vi "Tokenize Statement.vi"(8 "error in (no error)":errorcluster, 10 "Command":string) -> (0 "error out":errorcluster, 1 "Label":string, 2 "Arguments":string[](array[string]), 3 "Command":T1=enum."PASS", 4 "Label Arguments":string[](array[string]))   [LabVIEW 2023]
uses:
  Type Definitions/Command.ctl
  <vilib>/Utility/error.llb/Trim Whitespace One-Sided.vi
  <vilib>/Utility/error.llb/Error Cluster From Error Code.vi
  <vilib>/ErrorRing/Error Ring.xnode
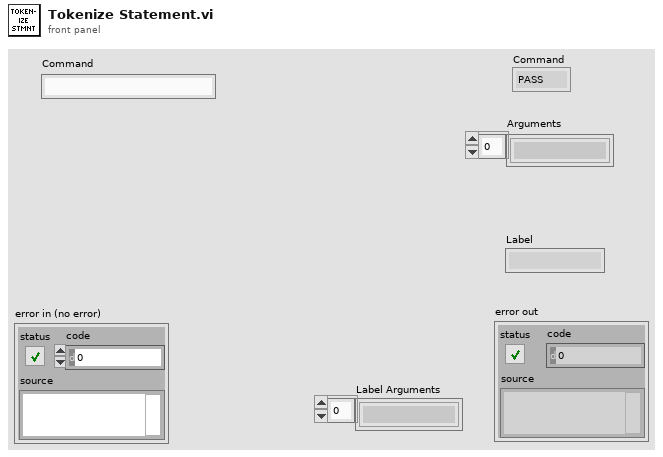
[diagram p1: front panel]
types:
  T1 = typedef "Command.ctl" = enum16{"", "PASS", "COPY", "PRINT", "GOTO", "GOTOIF", "GOTOIFN", "ADD", "SUB", "INC", "DEC", "HOME", "MOVEREL", "MOVENAME", "MOVETO", "GETPOS", "ROTATE", "GETROT", "SETVAC", "GETVAC", "JOYSTICK", "LOADTOOL", "UNLOADTOOL", "POTLINE", "POTDOT", "AUTOFOCUS", "FINDFID", "FIT", "WAIT", "MPGON", "MPGOFF", "PAUSE", "SNAPSHOT", "SETLOG", "CLEARLOG", "VIDEO", "TRANSFORMG2L", "TRANSFORML2G", "CHOICEPOPUP", "SETLIGHT", "CALL", "END", "DUMPSTATE", "FLEXREAD", "FLEXWRITE", "SURVEY", "LOADCONFIG", "SETERRORMODE", "COMPOSE", "INVERT", "EULER2QUAT", "QUAT2EULER", "MUL", "ROTATETO", "VERSION", "SIN", "COS", "TAN", "ATAN2", "ABS", "POW", "ACKFAULT", "MOVESAFE", "LOADSTAMP", "APPLYSTAMP", "UNLOADSTAMP", "LOADWEIGHT", "APPLYWEIGHT", "UNLOADWEIGHT", "RETURN", "GETFLOATPOPUP", "GETINTPOPUP", "GETVECPOPUP", "CLEARVARS", "PICKPART", "PLACEPART", "FITLINE", "XPRINT", "FITCIRCLE", "SAVESTATE", "DBLOGIN", "DBFINDCOMP", "DBLOGOUT", "DBSAVEASSEMBLY", "AEROSCRIPTRUN", "AEROSCRIPTSTOP", "AEROSCRIPTSTATUS", "DIALOG"}
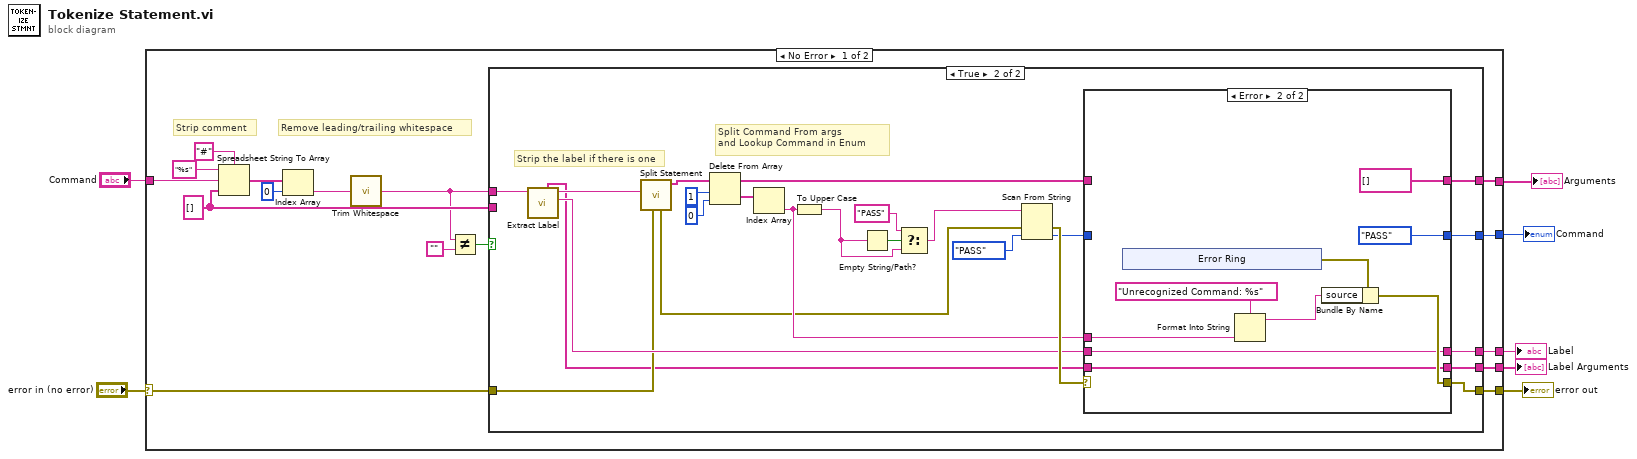
[diagram p0: block diagram]
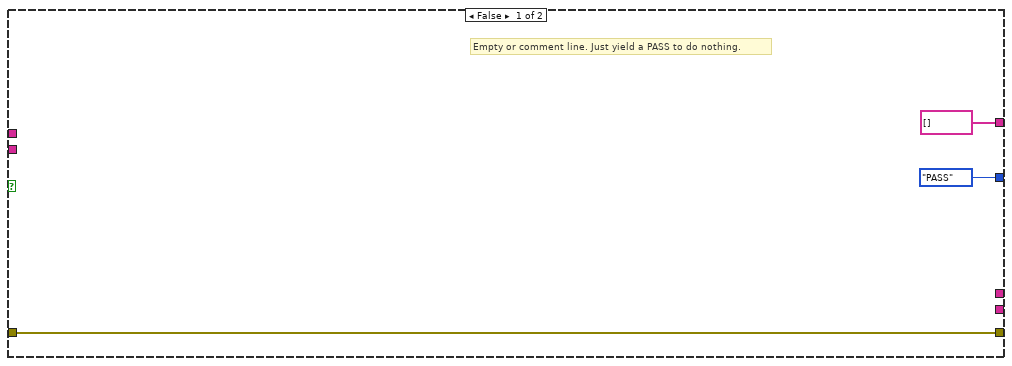
[diagram p2: hidden frame]
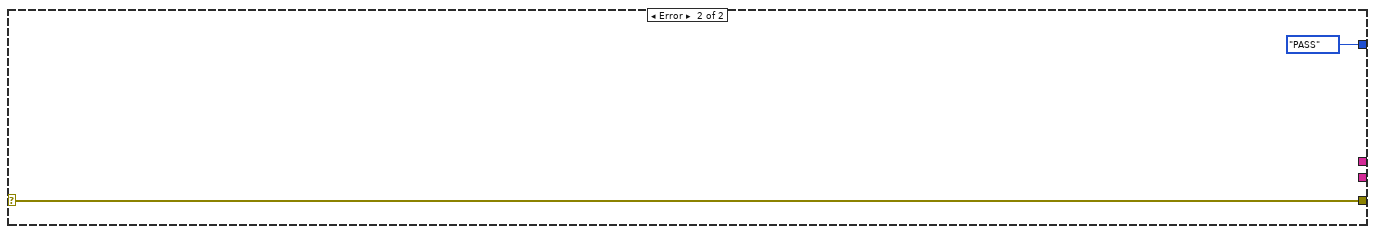
[diagram p4: hidden frame]
diagram:
  n1 = case shown="No Error" "error in (no error)" {
    selector: "error in (no error)" -> [w16 w69]
    tunnel: "Command" -> [w20 _]
    tunnel: [w13 _] -> w6
    tunnel: [w14 w69] -> w5
    tunnel: [w15 Command."PASS" ("Command 2")] -> w4
    tunnel: [w9 _] -> w2
    tunnel: [w8 _] -> w1
    frame No Error {
      w18 = string[] []
      # "Remove leading/trailing whitespace"
      # "Strip comment"
      n2 = Spreadsheet String To Array(delimiter (Tab)="#", format string="%s", spreadsheet string=w20, array type (2D Dbl)=w18) -> (array=w22:string[])
      n3 = Index Array(array=w22, index=0) -> (element=w19:string)
      n4 = call <vilib>:"Trim Whitespace.vi"("string"=w19) -> ("trimmed string"=w10:string)  [unwired: 1 in]
      n5 = Not Equal?(x=w10, y="") -> (x != y?=w12:bool)
      n6 = case shown="True" w12 {
        tunnel: w10 -> [_ w39]
        tunnel: w18 -> [_ _]
        tunnel: w16 -> [w24 w35]
        tunnel: [Command."PASS" ("Command 2") w44] -> w15
        tunnel: [w24 w43] -> w14
        tunnel: [string[] [] w41] -> w13
        tunnel: [_ w36] -> w9
        tunnel: [_ w27] -> w8
        frame False {
          # "Empty or comment line. Just yield a PASS to do nothing."
        }
        frame True {
          # "Strip the label if there is one"
          # "Split Command From args\nand Lookup Command in Enum"
          n7 = call "Extract Label.vi"("Statement in"=w39) -> ("Label"=w37:string, "Statement out"=w38:string, "Arguments"=w28:string[])  [unwired: 8 in]
          n8 = call "Split Statement.vi"("error in (no error)"=w35, "Statement"=w38) -> ("Tokens"=w40:string[], "error out"=w33:errorcluster)  [unwired: 8 in]
          n9 = Delete From Array(array=w40, length=1, index=0) -> (deleted portion=w48:string[], array with subset deleted=w42:string[])
          n10 = Index Array(array=w48) -> (element=w34:string)  [unwired: 1 in]
          n11 = To Upper Case(1:w34) -> (0:w30:string)
          n12 = Empty String/Path?(string/path=w30) -> (empty?=w32:bool)
          n13 = Select(t="PASS", s=w32, f=w30) -> (s? t:f=w29:string)
          n14 = Scan From String(input string=w29, error in=w33, default 1=Command."PASS" ("Command 2")) -> (error out=w46:errorcluster, output 1=w45:T1)  [unwired: 2 in, 2 out]
          n15 = case shown="Error" w46 {
            selector: w46 -> [w54 _]
            tunnel: w45 -> [w55 _]
            tunnel: [w55 Command."PASS" ("Command 2")] -> w44
            tunnel: [w54 w61] -> w43
            tunnel: w42 -> [w53 _]
            tunnel: [w53 string[] []] -> w41
            tunnel: w34 -> [_ w59]
            tunnel: w37 -> [w52 w57]
            tunnel: [w52 w57] -> w36
            tunnel: w28 -> [w51 w56]
            tunnel: [w51 w56] -> w27
            frame No Error {
            }
            frame Error {
              n16 = xnode "Error Ring"() -> ("error out"=w62:errorcluster)
              n17 = Format Into String(format string="Unrecognized Command: %s", w59) -> (resulting string=w58:string)  [unwired: 2 in, 1 out]
              n18 = Bundle By Name(cluster=w62, "source"=w58) -> (w61:errorcluster)
            }
          }
        }
      }
    }
    frame Error {
    }
  }
  "Arguments" <- w6
  "Command" <- w4
  "error out" <- w5
  "Label" <- w2
  "Label Arguments" <- w1
